vi "test_scp.vi"(9 "stop":bool) -> (0 "error out":errorcluster, 2 "manifold pressure":dbl)   [LabVIEW 2014]
panel:
  out "Numeric":i32
  out "standard error":string
  out "standard output":string
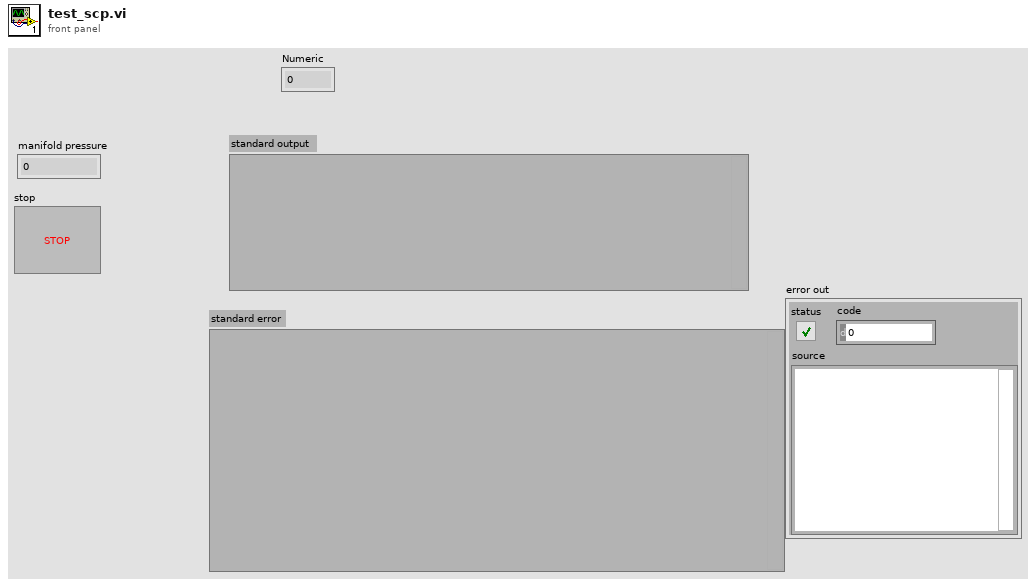
[diagram p1: front panel]
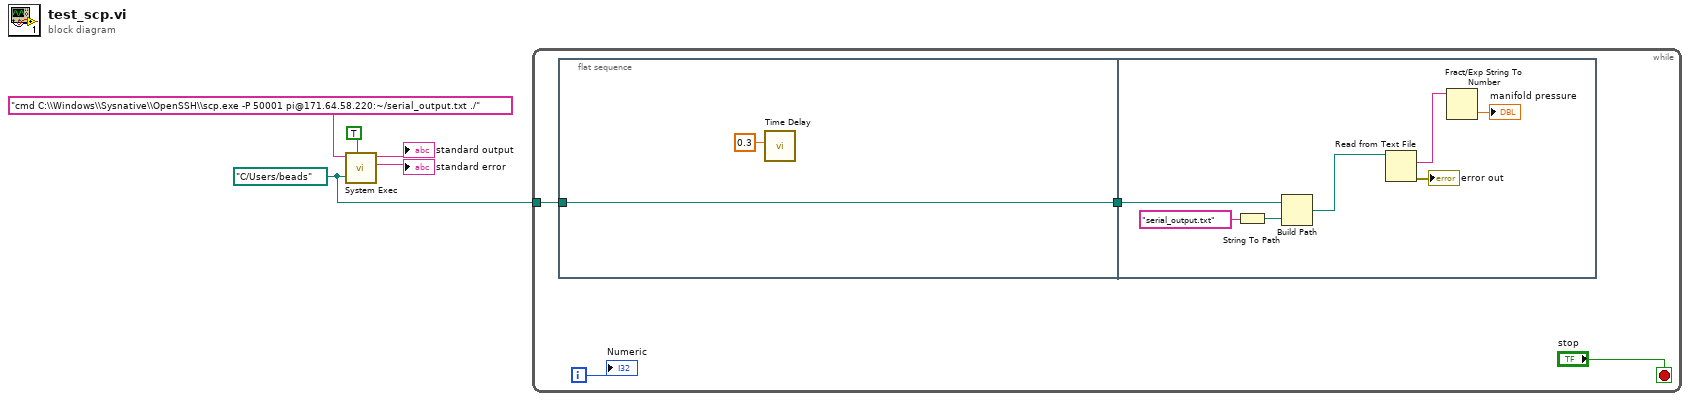
[diagram p0: block diagram]
diagram:
  w1 = path "C:/Users/beads" ("working directory")
  n1 = call <vilib>:"System Exec.vi"("wait until completion? (T)"=TRUE, "working directory"=w1, "command line"="cmd C:\\Windows\\Sysnative\\OpenSSH\\scp.exe -P 50001 pi@171.64.58.220:~/serial_output.txt ./") -> ("standard error"=→"standard error":string, "standard output"=→"standard output":string)  [unwired: 5 in, 2 out]
  n2 = while {
    tunnel: w1 -> [w6]
    i -> [w8]
    stop <- "stop" stop-if-true
    n3 = flat-sequence {
      tunnel: [w11] -> w7
      tunnel: w6 -> [w11]
      tunnel: w7 -> [w12]
      frame #0 {
        n4 = call "Time Delay"("Delay Time (s)"=0.3) -> ()  [unwired: 10 in, 1 out]
      }
      frame #1 {
        n5 = String To Path(string="serial_output.txt") -> (path=w17:path)
        n6 = Build Path(base path=w12, name or relative path=w17) -> (appended path=w16:path)
        n7 = Read from Text File(file (use dialog)=w16) -> (text=w15:string, error out=→"error out":errorcluster)  [unwired: 3 in, 2 out]
        n8 = Fract/Exp String To Number(string=w15) -> (number=→"manifold pressure":dbl)  [unwired: 3 in, 1 out]
      }
    }
    "Numeric" <- w8
  }
